vi "exemplo cluster erro.vi"() -> ()   [LabVIEW 2020]
panel:
  out "Dato capturado depois de ligar o dispositivo":dbl
  out "Dado antes de ligar o dispositivo":dbl
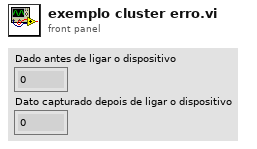
[diagram p1: front panel]
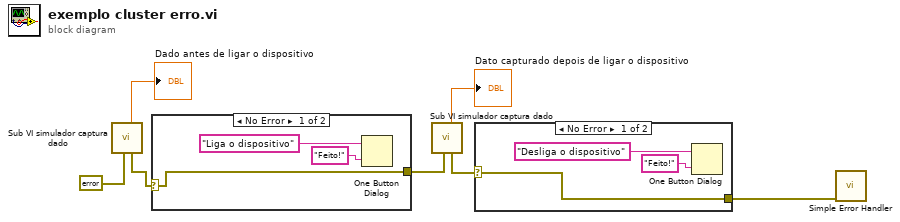
[diagram p0: block diagram]
diagram:
  n1 = call "Sub VI simulador captura dado.vi"("error constant"=errorcluster {"status"=FALSE, "code"=0, "source"=""}) -> ("error constant 2"=w2:errorcluster, "Dato capturado"=→"Dado antes de ligar o dispositivo":dbl)  [unwired: 9 in]
  n2 = case shown="No Error" w2 {
    selector: w2 -> [w8 w11]
    tunnel: [w8 w11] -> w5
    frame No Error {
      n3 = One Button Dialog(message="Liga o dispositivo", button name ("OK")="Feito!") -> ()  [unwired: 1 out]
    }
    frame Error {
    }
  }
  n4 = call "Sub VI simulador captura dado.vi"("error constant"=w5) -> ("error constant 2"=w7:errorcluster, "Dato capturado"=→"Dato capturado depois de ligar o dispositivo":dbl)  [unwired: 9 in]
  n5 = case shown="No Error" w7 {
    selector: w7 -> [w12 w15]
    tunnel: [w12 w15] -> w3
    frame No Error {
      n6 = One Button Dialog(message="Desliga o dispositivo", button name ("OK")="Feito!") -> ()  [unwired: 1 out]
    }
    frame Error {
    }
  }
  n7 = call <vilib>:"Simple Error Handler.vi"("error in (no error)"=w3) -> ()  [unwired: 4 in, 5 out]
